vi "ShooterSpeedRegulateV2 Debug.vi"() -> (4 "ALL GOOD":bool, 10 "Motor 1 Output":dbl)   [LabVIEW 2012]
uses:
  Robot Global Data.vi
  Max'sToolKit/ConvertVoltageToPercentVbs.vi
panel:
  in  "Shooter Speed":T1(ring)
  in  "Use PID":bool
  out "Waveform Chart":cluster{dbl, "upper limit":dbl, dbl}(graph)
  in  "Feed Foward \nVoltage":dbl format="%_6g"
  in  "PID gains":T2
  out "Motor Voltage":dbl
  out "Error":dbl
  in  "Reset Shooter PID":bool
  out "Loop Rate (Hz)":dbl
  out "Array Index":dbl
  out "Wheel 1 RPS":dbl
  out "W1 Target RPS":dbl
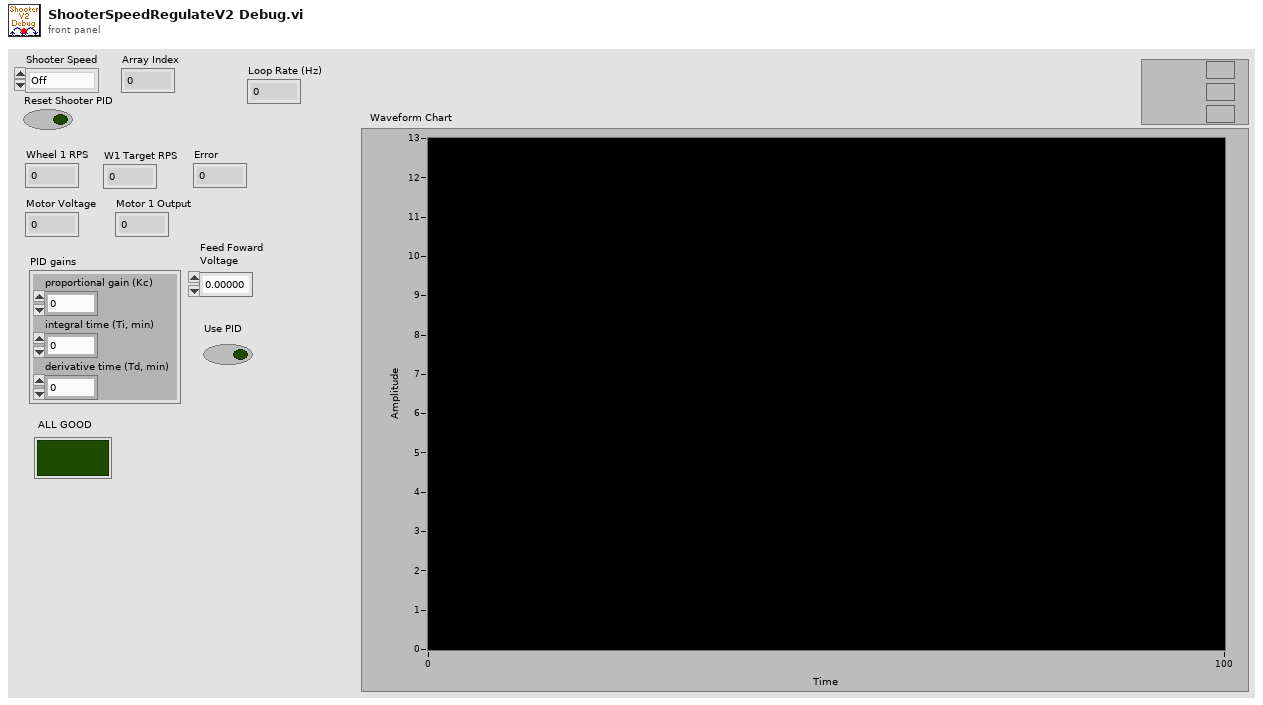
[diagram p1: front panel]
types:
  T1 = enum16{"Off", "Close Pyramid 3pt", "Far Pyramid 3pt", "Feeder Shot"}
  T2 = cluster{"proportional gain (Kc)":dbl, "integral time (Ti, min)":dbl, "derivative time (Td, min)":dbl}
  T3 = typedef "WPI_EncoderDevRef.ctl" = cluster{"DevStatus":errorcluster, "EncoderIndex":T4, "CounterIndex":T5, "DistancePerCount":dbl, "Decoding Type":T6}
  T4 = typedef "FPGA_EncoderIdx.ctl" = enum8{"Enc 0", "Enc 1", "Enc 2", "Enc 3", "Invalid"}
  T5 = typedef "FPGA_CounterCtrSystemIndex.ctl" = enum8{"Ctr 0", "Ctr 1", "Ctr 2", "Ctr 3", "Ctr 4", "Ctr 5", "Ctr 6", "Ctr 7", "Invalid"}
  T6 = typedef "WPI_EncoderType.ctl" = enum16{"1x", "2x", "4x"}
  T7 = typedef "WPI_MotorControlDeviceRef.ctl" = cluster{"DeviceStatus":errorcluster, "Type":enum16{"PWM", "CAN"}, "PWM":cluster{"Digital Module":T8, "PWM Channel":T9, "DeadBand":T10}, "CAN":cluster{"Device Number":u8, "Control Mode":T11, "Semaphore":T12, "Max Vout":dbl}, "Invert":bool, "TransformRef":T13, "InvTransformRef":T13}
  T8 = typedef "FPGA_TypedefDigitalModule.ctl" = enum16{"Digital Module 1", "Digital Module 2"}
  T9 = typedef "FPGA_DIOPWMChannel.ctl" = enum8{"PWM 1", "PWM 2", "PWM 3", "PWM 4", "PWM 5", "PWM 6", "PWM 7", "PWM 8", "PWM 9", "PWM 10", "Invalid"}
  T10 = typedef "WPI_PWMDeadband.ctl" = cluster{"Name":string, "maxPositivePwm":i32, "minPositivePwm":i32, "centerPwm":i32, "maxNegativePwm":i32, "minNegativePwm":i32, "angularRange":u16}
  T11 = typedef "WPI_CANJaguar_ControlMode.ctl" = enum8{"Percent VBus", "Current", "Speed", "Position", "Voltage"}
  T12 = typedef "Semaphore RefNum" = refnum<k1>
  T13 = typedef "WPI_PWMTransform_ConPane.ctl" = refnum<vi>
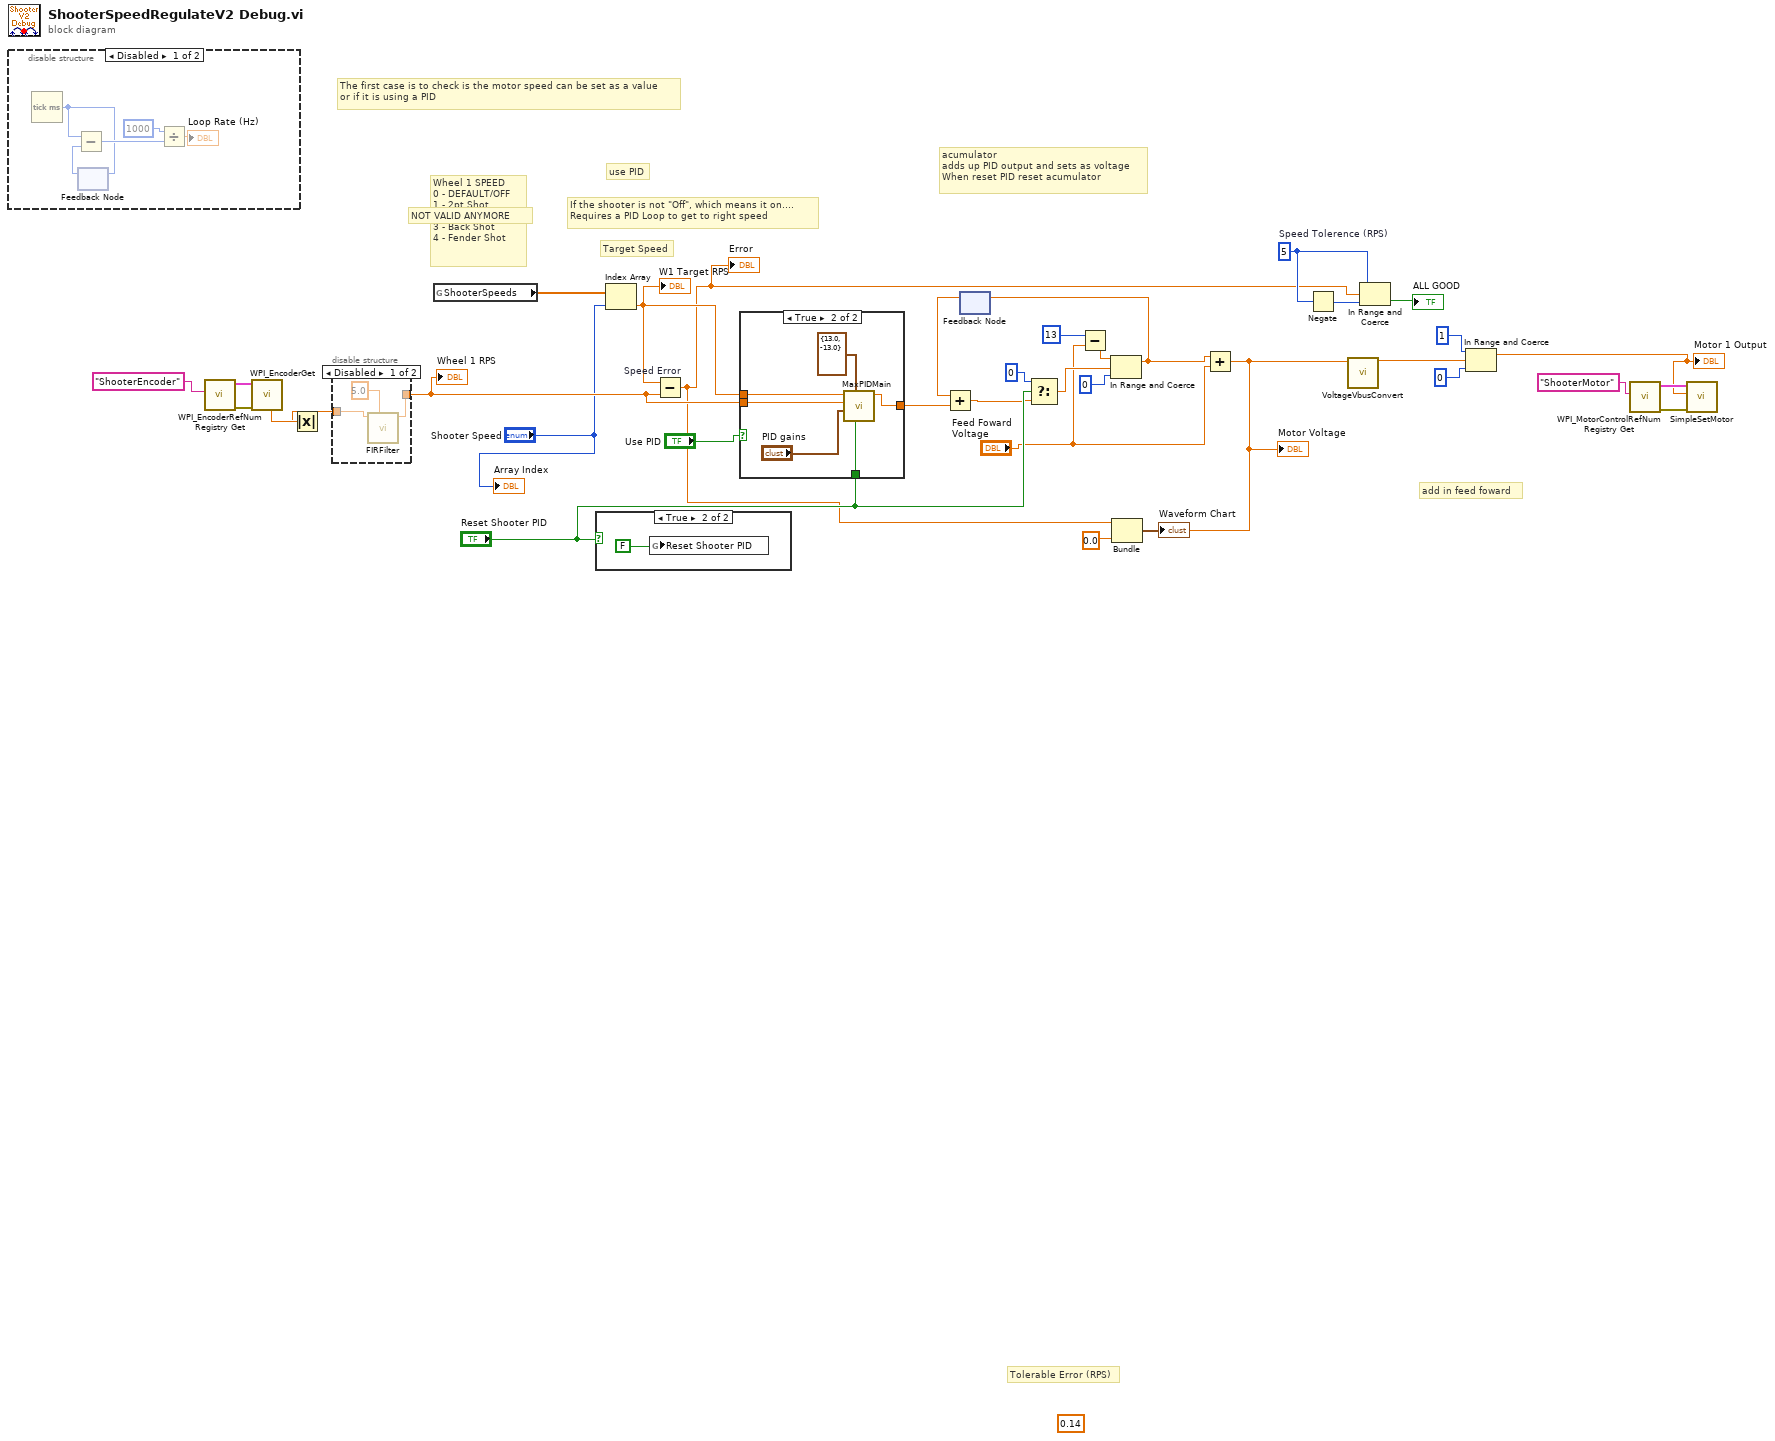
[diagram p0: block diagram]
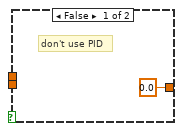
[diagram p2: hidden frame]
diagram:
  w22 = 5  # Speed Tolerence (RPS)
  (unwired) 0.14
  # "add in feed foward"
  # "acumulator\nadds up PID output and sets as voltage\nWhen reset PID reset acumulator"
  # "Target Speed"
  # "If the shooter is not \"Off\", which means it on....\nRequires a PID Loop to get to right speed"
  # "use PID"
  # "NOT VALID ANYMORE"
  # "The first case is to check is the motor speed can be set as a value\nor if it is using a PID"
  # "Tolerable Error (RPS)"
  # "Wheel 1 SPEED\n0 - DEFAULT/OFF\n1 - 2pt Shot\n2 - 3pt Key Shot\n3 - Back Shot\n4 - Fender Shot"
  n1 = disable-structure shown="Disabled" {
    frame Disabled {
      n2 = Tick Count (ms)() -> (millisecond timer value=w36:u32)
      n3 = feedback #1() -> (w37:u32)  [unwired: 1 in]
      n4 = Subtract(x=w36, y=w37) -> (x-y=w39:u32)
      n5 = feedback-in #1(w36) -> ()
      n6 = Divide(x=1000, y=w39) -> (x/y=→"Loop Rate (Hz)":dbl)
    }
    frame Enabled {
    }
  }
  n7 = call <vilib>:"WPI_EncoderRefNum Registry Get.vi"("refnum name"="ShooterEncoder") -> ("error out"=w29:errorcluster, "EncoderDevRef"=w30:T3)  [unwired: 9 in]
  n8 = call <vilib>:"WPI_EncoderGet.vi"("error in (no error)"=w29, "EncoderDevRef"=w30) -> ("Rate"=w26:dbl)  [unwired: 4 in, 5 out]
  n9 = Absolute Value(x=w26) -> (abs(x)=w25:dbl)
  n10 = disable-structure shown="Disabled" {
    disable-tunnel: [w42 w44] -> w28
    disable-tunnel: w25 -> [w41 w44]
    frame Disabled {
      n11 = call "FIRFilter.vi"("Filter Size"=5.0 ("Filter size"), "Input"=w41) -> ("Output"=w42:dbl)  [unwired: 9 in]
    }
    frame Enabled {
    }
  }
  "Wheel 1 RPS" <- w28
  n12 = global read "Robot Global Data.vi" "ShooterSpeeds"() -> (w27:dbl[])
  n13 = case shown="True" "Reset Shooter PID" {
    frame False {
    }
    frame True {
      n14 = global write "Robot Global Data.vi" "Reset Shooter PID"(FALSE) -> ()
    }
  }
  n15 = Index Array(array=w27, index="Shooter Speed") -> (element=w18:dbl)
  "W1 Target RPS" <- w18
  n16 = Subtract "Speed Error"(x=w18, y=w28) -> (x-y=w15:dbl)
  "Error" <- w15
  n17 = case shown="True" "Use PID" {
    tunnel: w28 -> [_ w52]
    tunnel: "Reset Shooter PID" -> [_ w51]
    tunnel: w18 -> [_ w48]
    tunnel: [0.0 ("output") w47] -> w17
    frame False {
      # "don't use PID"
    }
    frame True {
      n18 = call "MaxPIDMain.vi"("Reset"=w51, "Output Range"=cluster{"output high":dbl, "output low":dbl} {"output high"=13.0, "output low"=-13.0} ("output range"), "PID gains"="PID gains", "process variable"=w52, "setpoint"=w48) -> ("Output"=w47:dbl)  [unwired: 5 in, 1 out]
    }
  }
  n19 = feedback #2() -> (w19:dbl)  [unwired: 1 in]
  n20 = Add(x=w19, y=w17) -> (x+y=w11:dbl)
  n21 = Select(t=0, s="Reset Shooter PID", f=w11) -> (s? t:f=w16:dbl)
  n22 = Subtract(x=13 ("upper limit"), y="Feed Foward \nVoltage") -> (x-y=w9:dbl)
  n23 = In Range and Coerce(upper limit=w9, x=w16, lower limit=0 ("upper limit")) -> (coerced(x)=w8:dbl)  [unwired: 1 out]
  n24 = feedback-in #2(w8) -> ()
  n25 = Add(x=w8, y="Feed Foward \nVoltage") -> (x+y=w7:dbl)
  "Motor Voltage" <- w7
  n26 = Bundle(w15, w7, 0.0) -> (→"Waveform Chart":cluster{dbl, dbl, dbl})  [unwired: 1 in]
  n27 = Negate(x=w22) -> (-x=w32:i32)
  n28 = call-poly "VoltageVbusConvert.vi"("Voltage"=w7) -> ("Vbus"=w2:dbl)  [unwired: 10 in]
  n29 = In Range and Coerce(upper limit=w22, x=w15, lower limit=w32) -> (In Range?=→"ALL GOOD":bool)  [unwired: 1 out]
  n30 = In Range and Coerce(upper limit=1, x=w2, lower limit=0 ("upper limit")) -> (coerced(x)=w4:dbl)  [unwired: 1 out]
  "Motor 1 Output" <- w4
  n31 = call <vilib>:"WPI_MotorControlRefNum Registry Get.vi"("refnum name"="ShooterMotor") -> ("error out"=w33:errorcluster, "MotorControlDevRef"=w34:T7)  [unwired: 9 in]
  n32 = call "SimpleSetMotor.vi"("error in (no error)"=w33, "Output"=w4, "MotorControlDevRef"=w34) -> ()  [unwired: 7 in, 2 out]
  "Array Index" <- "Shooter Speed"
